vi "Encoder to 360.vi"(4 "Rear Right Data":T1, 5 "Rear Left Data":T1, 6 "Front Left Data":T1, 7 "Front Right Data":T1) -> (0 "Rear Right Data":T1, 1 "Rear Left Data":T1, 2 "Front Left Data":T1, 3 "Front Right Data":T1)   [LabVIEW 2018]
uses:
  Final Motor Data.ctl
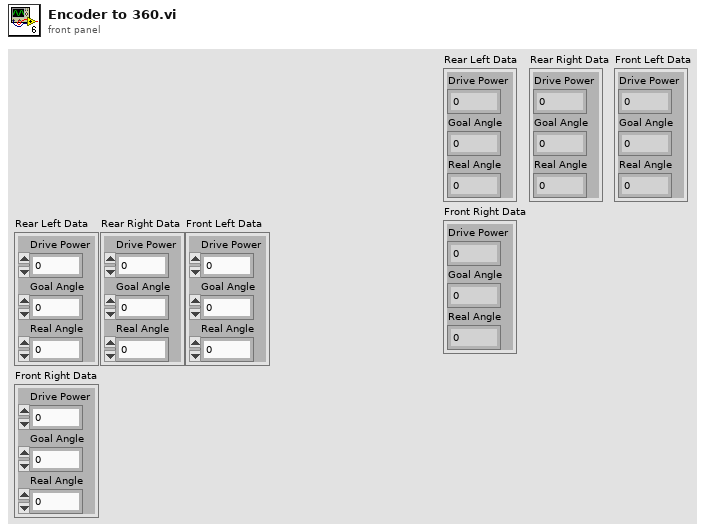
[diagram p1: front panel]
types:
  T1 = typedef "Final Motor Data.ctl" = cluster{"Drive Power":dbl, "Goal Angle":dbl, "Real Angle":dbl}
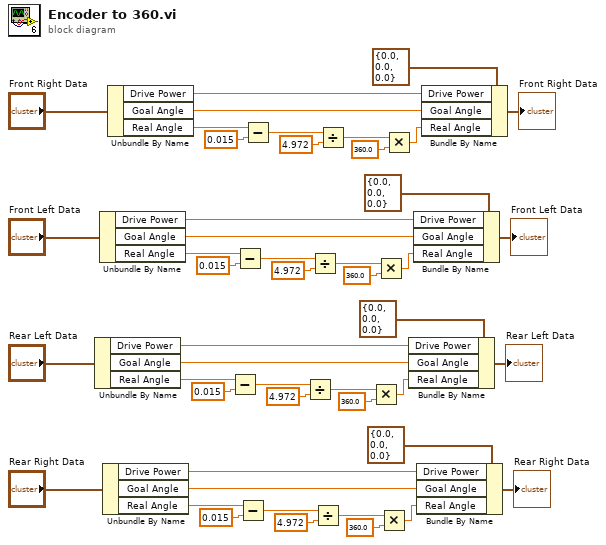
[diagram p0: block diagram]
diagram:
  n1 = Unbundle By Name("Rear Left Data") -> ("Drive Power"=w34:dbl, "Goal Angle"=w33:dbl, "Real Angle"=w4:dbl)
  n2 = Unbundle By Name("Front Left Data") -> ("Drive Power"=w32:dbl, "Goal Angle"=w31:dbl, "Real Angle"=w6:dbl)
  n3 = Unbundle By Name("Rear Right Data") -> ("Drive Power"=w36:dbl, "Goal Angle"=w35:dbl, "Real Angle"=w2:dbl)
  n4 = Unbundle By Name("Front Right Data") -> ("Drive Power"=w30:dbl, "Goal Angle"=w29:dbl, "Real Angle"=w8:dbl)
  n5 = Subtract(x=w4, y=0.015) -> (x-y=w17:dbl)
  n6 = Subtract(x=w6, y=0.015) -> (x-y=w22:dbl)
  n7 = Subtract(x=w2, y=0.015) -> (x-y=w12:dbl)
  n8 = Subtract(x=w8, y=0.015) -> (x-y=w27:dbl)
  n9 = Divide(x=w17, y=4.972) -> (x/y=w15:dbl)
  n10 = Divide(x=w22, y=4.972) -> (x/y=w20:dbl)
  n11 = Divide(x=w12, y=4.972) -> (x/y=w10:dbl)
  n12 = Divide(x=w27, y=4.972) -> (x/y=w25:dbl)
  n13 = Multiply(x=w15, y=360.0) -> (x*y=w3:dbl)
  n14 = Multiply(x=w20, y=360.0) -> (x*y=w5:dbl)
  n15 = Multiply(x=w10, y=360.0) -> (x*y=w1:dbl)
  n16 = Multiply(x=w25, y=360.0) -> (x*y=w7:dbl)
  n17 = Bundle By Name(cluster=T1 {"Drive Power"=0.0, "Goal Angle"=0.0, "Real Angle"=0.0} ("Data"), "Drive Power"=w34, "Goal Angle"=w33, "Real Angle"=w3) -> (→"Rear Left Data":T1)
  n18 = Bundle By Name(cluster=T1 {"Drive Power"=0.0, "Goal Angle"=0.0, "Real Angle"=0.0} ("Data"), "Drive Power"=w32, "Goal Angle"=w31, "Real Angle"=w5) -> (→"Front Left Data":T1)
  n19 = Bundle By Name(cluster=T1 {"Drive Power"=0.0, "Goal Angle"=0.0, "Real Angle"=0.0} ("Data"), "Drive Power"=w36, "Goal Angle"=w35, "Real Angle"=w1) -> (→"Rear Right Data":T1)
  n20 = Bundle By Name(cluster=T1 {"Drive Power"=0.0, "Goal Angle"=0.0, "Real Angle"=0.0} ("Data"), "Drive Power"=w30, "Goal Angle"=w29, "Real Angle"=w7) -> (→"Front Right Data":T1)
